vi "KE622x -- Get Current Level.vi"(0 "Resource In":refnum<visa-resource-name>, 1 "Check For SCPI Errors? (T)":bool=TRUE, 11 "error in (no error)":errorcluster) -> (4 "Resource Out (dupl)":refnum<visa-resource-name>, 8 "Current Level (A)":dbl=0.1 min=-0.105 max=0.105 format="%.4p", 15 "error out":errorcluster)   [LabVIEW 2013, in "Keithly user program.lvlib"]
doc: "Returns the output current level when the source is operating in a DC mode (i.e. static mode)."
uses:
  Keithly user program.lvlib
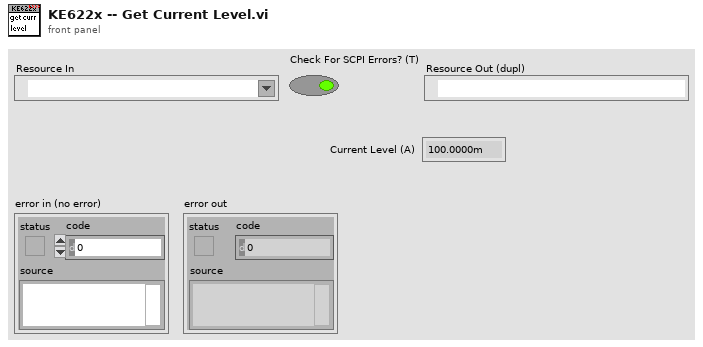
[diagram p1: front panel]
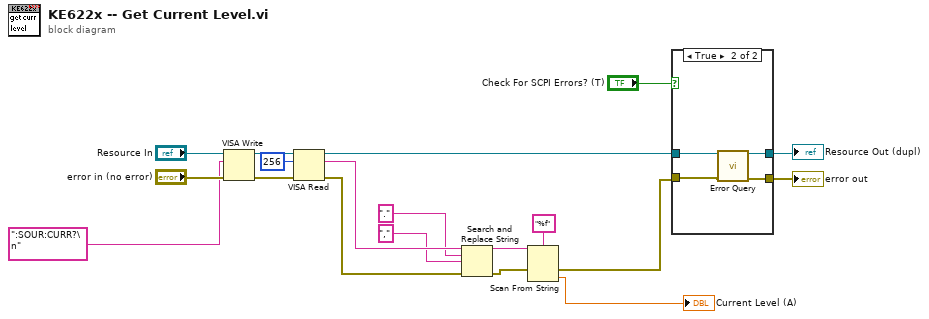
[diagram p0: block diagram]
diagram:
  n1 = VISA Write(VISA resource name="Resource In", write buffer=":SOUR:CURR?\n" ("format string"), error in (no error)="error in (no error)") -> (VISA resource name out=w13:refnum<visa-resource-name>, error out=w12:errorcluster)  [unwired: 1 out]
  n2 = VISA Read(VISA resource name=w13, byte count=u32 256, error in (no error)=w12) -> (VISA resource name out=w8:refnum<visa-resource-name>, read buffer=w4:string, error out=w3:errorcluster)  [unwired: 1 out]
  n3 = Search and Replace String(input string=w4, search string=".", replace string="," ("replace string (\"\")"), error in=w3) -> (result string=w6:string, error out=w5:errorcluster)  [unwired: 4 in, 2 out]
  n4 = Scan From String(format string="%f", input string=w6, error in=w5) -> (error out=w9:errorcluster, output 1=→"Current Level (A)":dbl)  [unwired: 2 in, 2 out]
  n5 = case shown="True" "Check For SCPI Errors? (T)" {
    tunnel: w8 -> [w21 w24]
    tunnel: w9 -> [w20 w23]
    tunnel: [w20 w22] -> w15
    tunnel: [w21 w25] -> w16
    frame False {
    }
    frame True {
      n6 = call "Error Query.vi"("VISA Resource In"=w24, "error in (no error)"=w23) -> ("VISA Resource Out (dupl)"=w25:refnum<visa-resource-name>, "error out"=w22:errorcluster)  [unwired: 10 in, 2 out]
    }
  }
  "Resource Out (dupl)" <- w16
  "error out" <- w15
